vi "Actor Core.vi"(8 "error in (no error)":errorcluster, 11 "Waveform Plot.lvclass":refnum<class "Waveform Plot.lvclass">) -> (0 "error out":errorcluster, 3 "Actor out":refnum<class "Actor.lvclass">)   [LabVIEW 2015, in "Waveform Plot.lvclass"]
doc: "<B>Copyright:</B> (c) 2015 National Instruments. All rights reserved.\n\nOpens the .tdms file specified in the <B>file path</B> input and presents the file data in the TDMS File Viewer dialog box."
uses:
  Waveform Plot.lvclass
  Instance           1 26Saved   TDMS - File Viewer .vi
  <vilib>/Utility/tdmsutil.llb/fileViewerConfigData.ctl
  <vilib>/Utility/tdmsutil.llb/TDMSFileViewerLocalizedText.vi
  <vilib>/Utility/error.llb/DialogType.ctl
  <vilib>/event_ctls.llb/sizeaction.ctl
  <vilib>/event_ctls.llb/panelstate.ctl
  Plot/Plot.lvclass
  <vilib>/ActorFramework/Actor/Actor.lvclass
panel:
  out "LastXScaleFormat":u8
  out "TotalCount":u64
  out "Temp Configuration":T1
  in  "LastTopLeftValue":u64
  out "Resize?":bool
  in  "Help":bool
  out "file path out":path
  in  "Status":string
  in  "Settings...":bool
  in  "file path":path
  in  "Properties / Values / Graph":T2(tab)=enum."Analog values (graph)"
  in  "Properties":i32(listbox)
  in  "Quit":bool
  in  "Go To":bool
  in  "Scrollbar":u64(c297)
  in  "Raw data values":i32(listbox)
  out "Waveform Graph":waveform(dbl)[](graph)
  in  "File contents":string(tree)
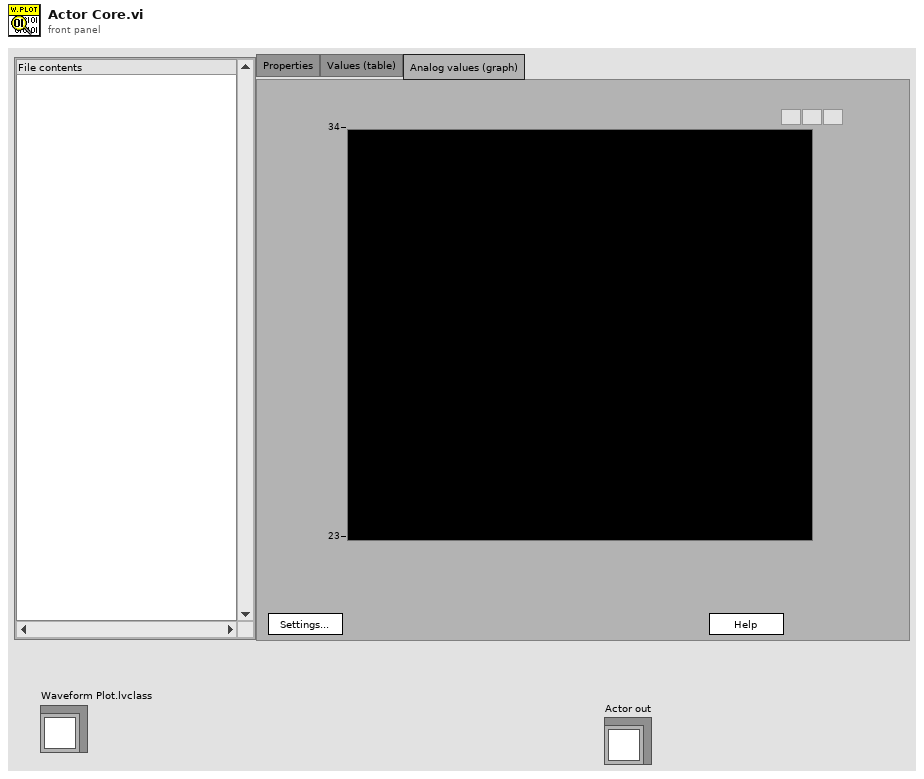
[diagram p1: front panel]
types:
  T1 = typedef "fileViewerConfigData.ctl" = cluster{"Show all (table)":bool, "Show all (graph)":bool, "limit (table)":u64, "limit (graph)":u64, "no show":bool, "start (table)":u64, "start (graph)":u64}
  T2 = enum32{"Properties", "Values (table)", "Analog values (graph)"}
  T3 = enum16{"open", "open or create", "create or replace", "create", "open (read-only)"}
  T4 = cluster{"Tree":refnum<vi>, "Tab Control":refnum<vi>, "property list":refnum<vi>, "raw data list":refnum<vi>, "Waveform Graph":refnum<vi>, "Ok":refnum<vi>, "Ok 2":refnum<vi>, "Ok 3":refnum<vi>, "Ok 4":refnum<vi>, "Scrollbar":refnum<vi>, "Ok 5":refnum<vi>, "TopLeftValue":refnum<vi>, "TotalCount":refnum<vi>}
  T5 = cluster{"File Path Control":path, "Group":string, "Channel":string, "Abbreviated":string}[]
  T6 = cluster{"File Path Control":path, "Group":string, "Channel":string, "Abbreviated":string}
  T7 = typedef "panelstate.ctl" = enum32{"Standard", "Minimized", "Maximized"}
  T8 = typedef "sizeaction.ctl" = enum32{"Minimized", "Maximized", "Resized"}
  T9 = cluster{"Shift":bool, "Ctrl":bool, "Alt":bool, "Cmd":bool, "Opt":bool}
  T10 = typedef "LVRectTypeDef.ctl" = cluster{"Left":i16, "Top":i16, "Right":i16, "Bottom":i16}
  T11 = typedef "LVRowAndColumnUnsignedTypeDef.ctl" = cluster{"Row":u32, "Column":u32}
  T12 = typedef "DialogType.ctl" = u16
  T13 = typedef "eventvkey.ctl" = enum16{"ASCII", "Enter", "Return", "Shift", "Ctrl", "Alt", "Cmd", "Opt", "Caps", "NumLock", "Clear", "Break", "Up", "Down", "Left", "Right", "Insert", "Delete", "Home", "End", "PageUp", "PageDown", "Escape", "Help", "Pause", "ScrollLock", "F1", "F2", "F3", "F4", "F5", "F6", "F7", "F8", "F9", "F10", "F11", "F12", "F13", "F14", "F15", "F16", "F17", "F18", "F19", "F20", "F21", "F22", "F23", "F24", "Play", "VolumeUp", "VolumeDown", "Mute", "Two Byte Char"}
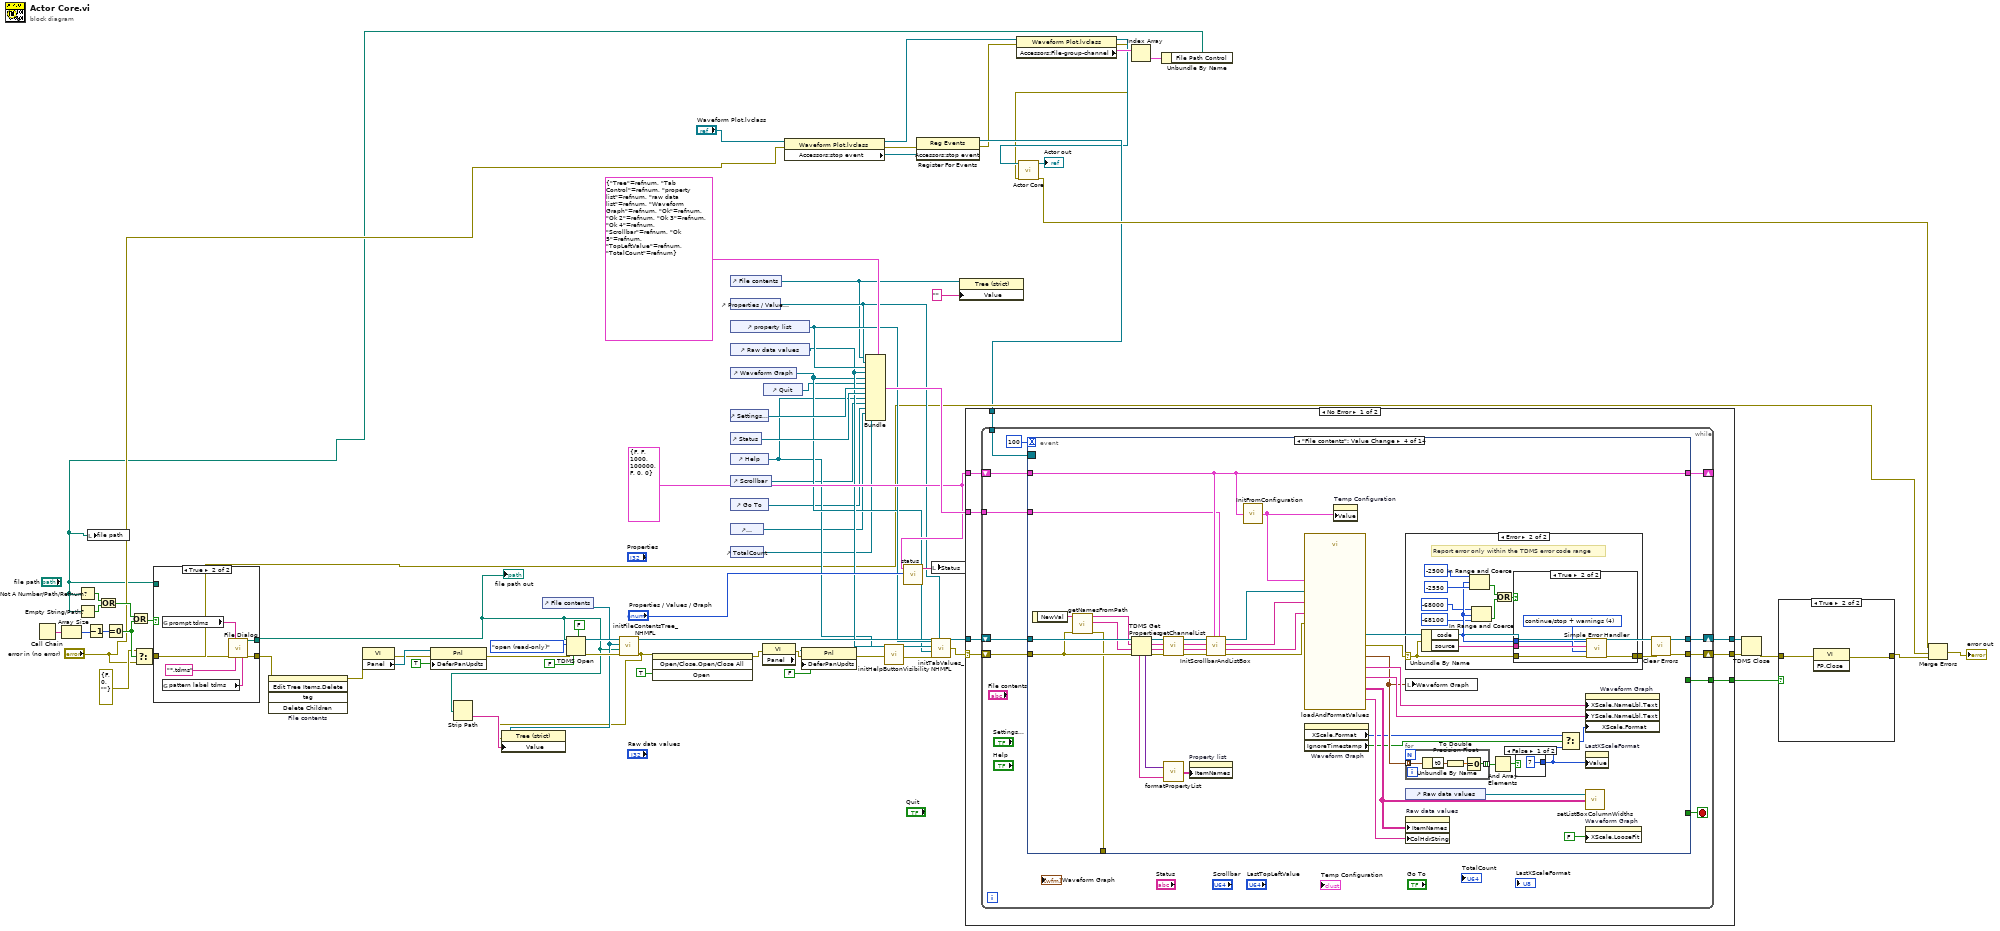
[diagram p0: block diagram]
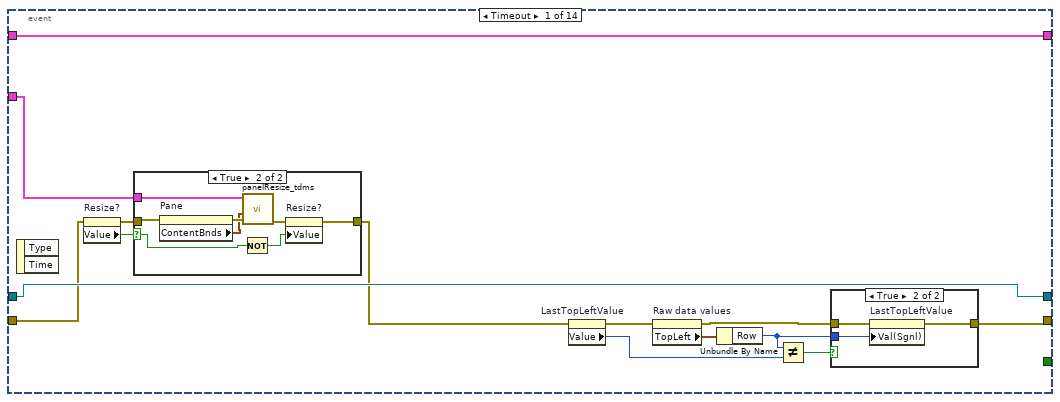
[diagram p3: hidden frame]
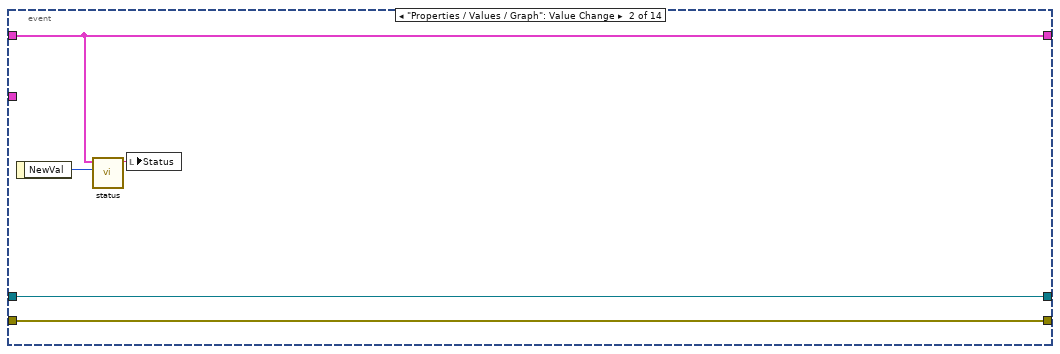
[diagram p6: hidden frame]
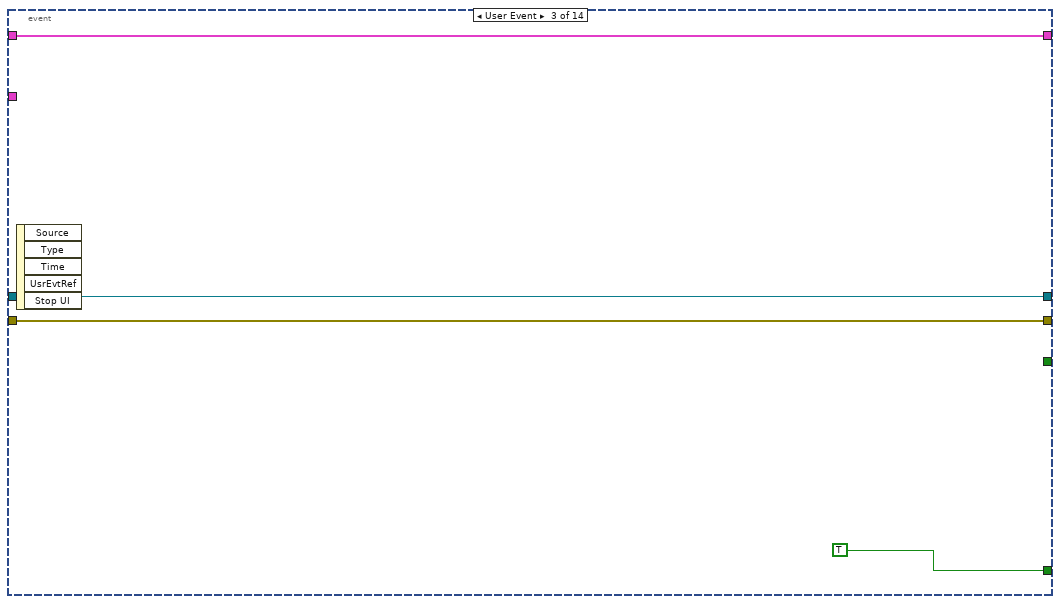
[diagram p7: hidden frame]
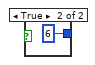
[diagram p8: hidden frame]
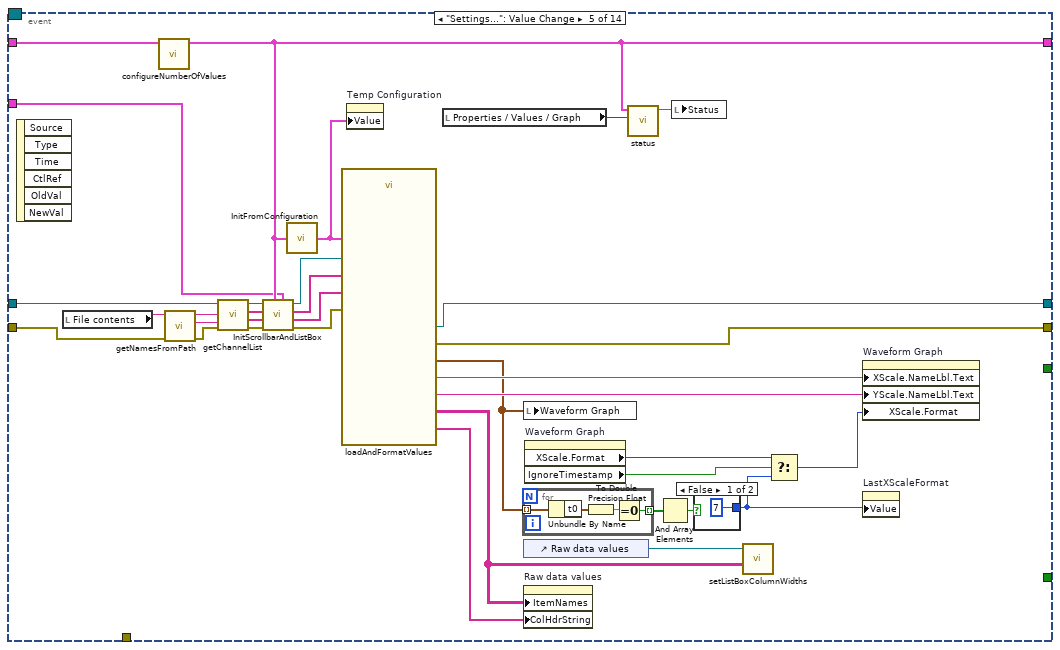
[diagram p11: hidden frame]
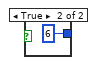
[diagram p12: hidden frame]
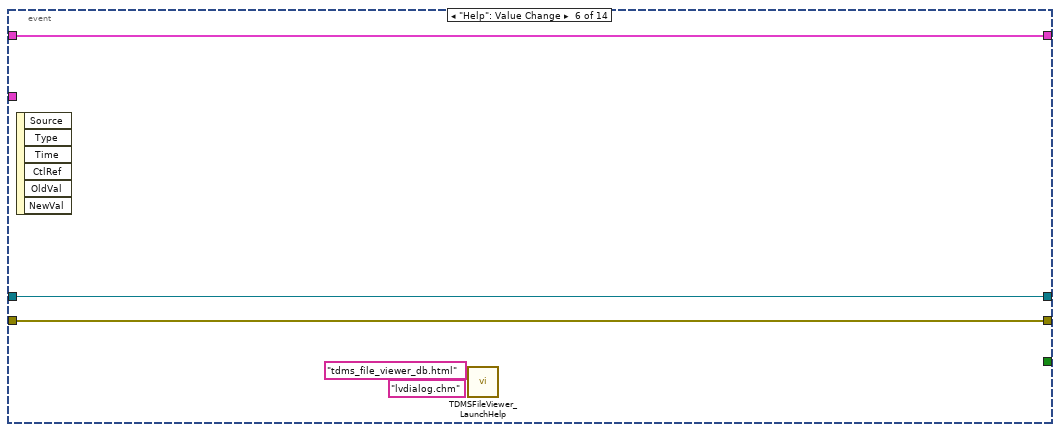
[diagram p13: hidden frame]
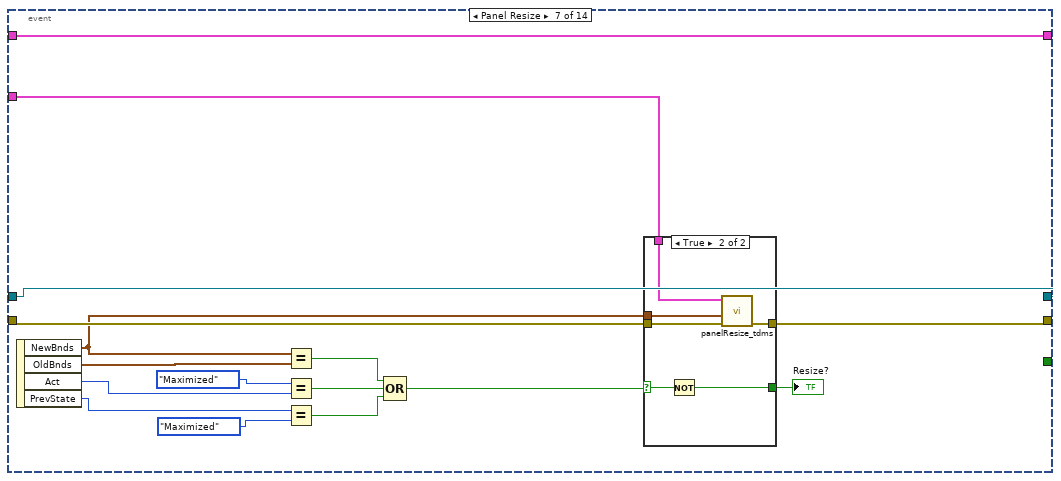
[diagram p14: hidden frame]
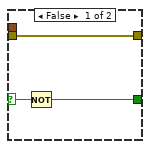
[diagram p15: hidden frame]
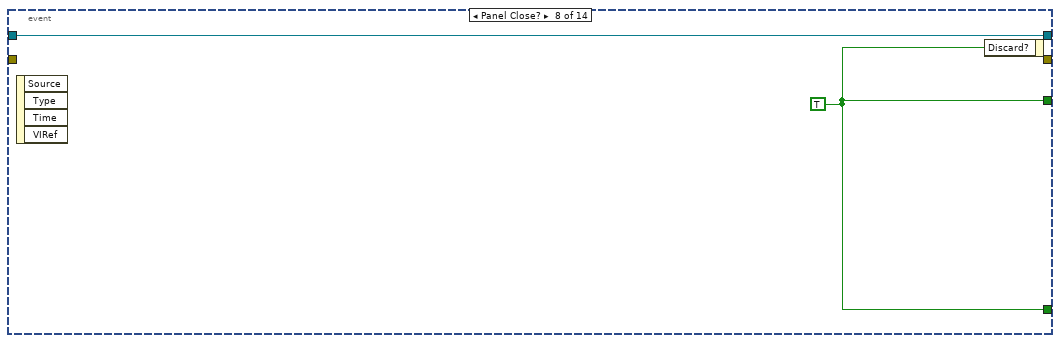
[diagram p16: hidden frame]
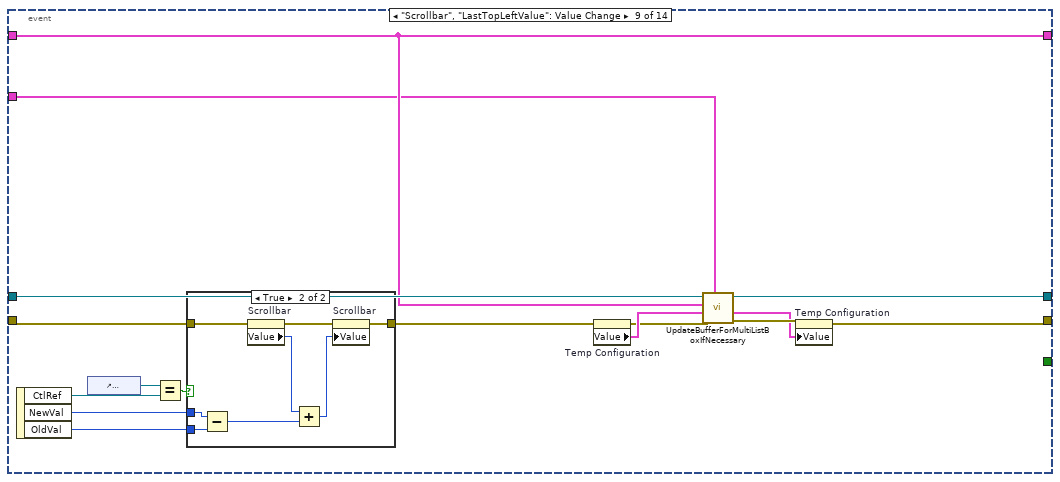
[diagram p17: hidden frame]
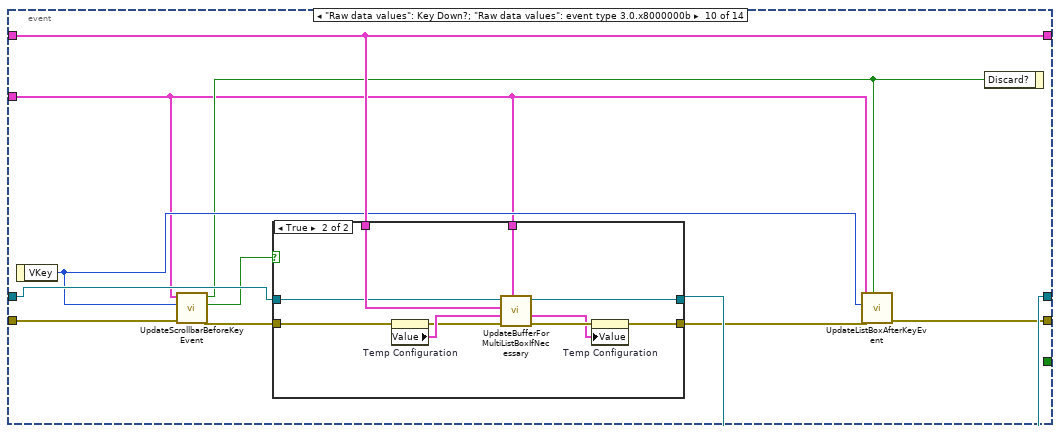
[diagram p19: hidden frame]
diagram:
  w44 = T1 {"Show all (table)"=FALSE, "Show all (graph)"=FALSE, "limit (table)"=1000, "limit (graph)"=100000, "no show"=FALSE, "start (table)"=0, "start (graph)"=0} ("TDMS File Viewer Configuration")
  n1 = Call Chain() -> (call chain=w56:string[])
  n2 = Array Size(array=w56) -> (size(s)=w54:i32)
  n3 = Decrement(x=w54) -> (x-1=w53:i32)
  n4 = Equal To 0?(x=w53) -> (x = 0?=w42:bool)
  n5 = Select(t=errorcluster {"status"=FALSE, "code"=0, "source"=""}, s=w42, f="error in (no error)") -> (s? t:f=w25:errorcluster)
  n6 = control-ref of="File contents"() -> (w4:refnum<vi>)
  n7 = control-ref of="File contents"() -> (w32:refnum<vi>)
  n8 = control-ref of="Properties / Values / Graph"() -> (w33:refnum<vi>)
  n9 = control-ref of="property list"() -> (w36:refnum<vi>)
  n10 = control-ref of="Raw data values"() -> (w35:refnum<vi>)
  n11 = control-ref of="Waveform Graph"() -> (w34:refnum<vi>)
  n12 = control-ref of="Settings..."() -> (w49:refnum<vi>)
  n13 = control-ref of="Status"() -> (w46:refnum<vi>)
  n14 = control-ref of="Help"() -> (w28:refnum<vi>)
  n15 = control-ref of="Scrollbar"() -> (w24:refnum<vi>)
  n16 = control-ref of="Go To"() -> (w23:refnum<vi>)
  n17 = control-ref of="LastTopLeftValue"() -> (w22:refnum<vi>)
  n18 = control-ref of="TotalCount"() -> (w21:refnum<vi>)
  n19 = control-ref of="Quit"() -> (w6:refnum<vi>)
  n20 = property class="Waveform Plot.lvclass"(reference="Waveform Plot.lvclass", error in="error in (no error)") -> (reference out=w10:refnum<class "Waveform Plot.lvclass">, error out=w15:errorcluster, "Accessors:stop event"=w14:refnum<user-event>)
  n21 = Bundle(cluster=T4 {"Tree"=refnum, "Tab Control"=refnum, "property list"=refnum, "raw data list"=refnum, "Waveform Graph"=refnum, "Ok"=refnum, "Ok 2"=refnum, "Ok 3"=refnum, "Ok 4"=refnum, "Scrollbar"=refnum, "Ok 5"=refnum, "TopLeftValue"=refnum, "TotalCount"=refnum} ("control refs"), "Tree"=w32, "Tab Control"=w33, "property list"=w36, "raw data list"=w35, "Waveform Graph"=w34, "Ok"=w6, "Ok 2"=w49, "Ok 3"=w46, "Ok 4"=w28, "Scrollbar"=w24, "Ok 5"=w23, "TopLeftValue"=w22, "TotalCount"=w21) -> (w51:T4)
  n22 = call <vilib>:"status.vi"("tab sheet"="Properties / Values / Graph", "TDMS File Viewer Configuration"=w44) -> ("status"=w45:string)  [unwired: 5 out]
  n23 = register-events(error in=w15, w14) -> (reference out=w13:refnum<event-registration>, error out=w8:errorcluster)  [unwired: 1 in]
  n24 = local write "Status"(w45) -> ()
  n25 = property class="Tree (strict)"(reference=w32, "Value"="") -> ()  [unwired: 1 in, 2 out]
  n26 = property class="Waveform Plot.lvclass"(reference=w10, error in=w8) -> (reference out=w9:refnum<class "Waveform Plot.lvclass">, error out=w7:errorcluster, "Accessors:File-group-channel"=w11:T5)
  n27 = call-parent "Actor Core.vi"("error in"=w7, "Measure Object in"=w9) -> ("error out"=w17:errorcluster, "Actor out"=→"Actor out":refnum<class "Actor.lvclass">)  [unwired: 8 in]
  n28 = Index Array(array=w11) -> (element=w12:T6)  [unwired: 1 in]
  n29 = Unbundle By Name(w12) -> ("File Path Control"=w5:path)
  n30 = Not A Number/Path/Refnum?(number/path/refnum=w5) -> (NaN/Path/Refnum?=w58:bool)
  n31 = Empty String/Path?(string/path=w5) -> (empty?=w57:bool)
  n32 = local write "file path"(w5) -> ()
  n33 = Or(x=w58, y=w57) -> (x .or. y?=w55:bool)
  n34 = Or(x=w55, y=w42) -> (x .or. y?=w52:bool)
  n35 = case shown="True" w52 {
    tunnel: [w75 w81] -> w3
    tunnel: w5 -> [w75 _]
    tunnel: [w74 w79] -> w47
    tunnel: w25 -> [w74 w78]
    frame False {
    }
    frame True {
      n36 = global read "TDMSFileViewerLocalizedText.vi" "prompt tdms"() -> (w77:string)
      n37 = global read "TDMSFileViewerLocalizedText.vi" "pattern label tdms"() -> (w76:string)
      n38 = call "File Dialog"("prompt"=w77, "error in"=w78, "pattern (all files)"="*.tdms", "pattern label"=w76) -> ("selected path"=w81:path, "error out"=w79:errorcluster)  [unwired: 3 in, 7 out]
    }
  }
  "file path out" <- w3
  n39 = invoke on="File contents" class="Tree (strict)" method="Edit Tree Items.Delete"(error in=w47) -> (error out=w64:errorcluster)  [unwired: 4 in, 4 out]
  n40 = property class="VI"(error in=w64) -> (error out=w65:errorcluster, "Panel"=w66:refnum<vi>)  [unwired: 1 in, 1 out]
  n41 = property class="Pnl"(reference=w66, error in=w65, "DeferPanUpdts"=TRUE ("Defer Panel Updates")) -> (error out=w68:errorcluster)  [unwired: 1 out]
  n42 = Strip Path(path=w3) -> (name=w2:string)  [unwired: 1 out]
  n43 = TDMS Open(5:FALSE ("create index file? (T)"), 6:FALSE ("disable buffering (T)"), 8:w68, 10:T3."open (read-only)" ("operation"), 11:w3) -> (0:w73:errorcluster, 3:w72:refnum<k34>)  [unwired: 2 in]
  n44 = call "initFileContentsTree_NHMFL.vi"("error in (no error)"=w73, "file path"=w3, "Tree Refnum"=w4, "tdms file"=w72) -> ("error out"=w1:errorcluster, "tdms file out"=w71:refnum<k34>)  [unwired: 2 out]
  n45 = property class="Tree (strict)"(reference=w4, error in=w1, "Value"=w2) -> ()  [unwired: 2 out]
  n46 = invoke on="File contents" class="Tree (strict)" method="Open/Close.Open/Close All"(error in=w1, "Open"=TRUE ("Open?")) -> (error out=w60:errorcluster)  [unwired: 2 in, 3 out]
  n47 = property class="VI"(error in=w60) -> (error out=w62:errorcluster, "Panel"=w61:refnum<vi>)  [unwired: 1 in, 1 out]
  n48 = property class="Pnl"(reference=w61, error in=w62, "DeferPanUpdts"=FALSE ("Defer Panel Updates")) -> (error out=w30:errorcluster)  [unwired: 1 out]
  n49 = call <vilib>:"initHelpButtonVisibility.vi"("error in"=w30, "Help"=w28) -> ("error out"=w29:errorcluster)  [unwired: 9 in]
  n50 = call "initTabValues_NHMFL.vi"("properties"=w36, "Values"=w35, "waveform"=w34, "error in"=w29, "Properties / Values / Graph"=w33) -> ("error out"=w37:errorcluster)
  n51 = case shown="No Error" w37 {
    selector: w37 -> [w84 w407]
    tunnel: w71 -> [w89 w408]
    tunnel: [w88 w408] -> w70
    tunnel: [w87 w406] -> w69
    tunnel: w51 -> [w86 _]
    tunnel: w44 -> [w85 _]
    tunnel: [w83 FALSE] -> w40
    tunnel: w13 -> [w82 _]
    frame No Error {
      n52 = while {
        shift-right: [w98] -> w87
        shift-left: w84 -> [w99]
        shift-right: [w97] -> w88
        shift-left: w89 -> [w100]
        tunnel: w86 -> [w95]
        shift-right: [w93] -> _
        shift-left: w85 -> [w94]
        tunnel: [w92] -> w83
        tunnel: w82 -> [w90]
        stop <- w96 stop-if-true
        n53 = event shown="[3] \"File contents\": Value Change" {
          selector: w90 -> [_ _ _ _ _ _ _ _ _ _ _ _ _ _]
          dyn-events: _ -> [_ _ _ _ _ _ _ _ _ _ _ _ _ _]
          timeout: 100 -> [_ _ _ _ _ _ _ _ _ _ _ _ _ _]
          tunnel: w100 -> [w114 w131 w135 w177 w225 w245 w262 w273 w289 w308 w333 w348 w381 w398]
          tunnel: w99 -> [w109 w132 w134 w169 w232 w244 w260 _ w276 w300 w322 w345 w380 w397]
          tunnel: [w102 w132 w134 w165 w233 w244 w259 _ w283 w305 w325 w346 w380 w389] -> w98
          tunnel: [w114 w131 w135 w176 w234 w245 w262 w273 w288 w307 w332 w347 w381 w398] -> w97
          tunnel: [_ _ TRUE ("Quit") _ _ _ _ w272 _ _ _ _ _ _] -> w96
          tunnel: [_ _ _ w168 _ _ _ _ _ _ _ _ _ _] -> _
          tunnel: w95 -> [w110 _ _ w144 w209 _ w261 _ w275 w301 w323 w342 _ _]
          tunnel: w94 -> [w113 w128 w133 w145 w235 w246 w258 _ w287 w309 w334 w349 w382 w399]
          tunnel: [w113 w128 w133 w145 w211 w246 w258 _ w287 w309 w334 w349 w382 w399] -> w93
          tunnel: [_ _ _ _ _ _ _ w272 _ _ _ _ _ _] -> w92
          event Timeout {
            n54 = event-data() -> ()  [unwired: 3 out]
            n55 = property on="Resize?" class="Bool (strict)"(error in=w109) -> (error out=w111:errorcluster, "Value"=w112:bool)  [unwired: 1 in, 1 out]
            n56 = case shown="True" w112 {
              selector: w112 -> [_ w126]
              tunnel: w110 -> [_ w127]
              tunnel: w111 -> [w119 w122]
              tunnel: [w119 w124] -> w107
              frame False {
              }
              frame True {
                n57 = property on="Pane" class="Pane"(error in=w122) -> (error out=w121:errorcluster, "ContentBnds"=w120:T10)  [unwired: 1 in, 1 out]
                n58 = Not(x=w126) -> (.not. x?=w123:bool)
                n59 = call <vilib>:"panelResize_tdms.vi"("error in (no error)"=w121, "NewBnds"=w120, "control refs"=w127) -> ("error out"=w125:errorcluster)  [unwired: 4 in]
                n60 = property on="Resize?" class="Bool (strict)"(error in=w125, "Value"=w123) -> (error out=w124:errorcluster)  [unwired: 1 in, 1 out]
              }
            }
            n61 = property on="LastTopLeftValue" class="DigNum (strict)"(error in=w107) -> (error out=w106:errorcluster, "Value"=w105:u64)  [unwired: 1 in, 1 out]
            n62 = property on="Raw data values" class="MCListbox (strict)"(error in=w106) -> (error out=w103:errorcluster, "TopLeft"=w108:T11)  [unwired: 1 in, 1 out]
            n63 = Unbundle By Name(w108) -> ("Row"=w101:u32)
            n64 = Not Equal?(x=w101, y=w105) -> (x != y?=w104:bool)
            n65 = case shown="True" w104 {
              tunnel: w103 -> [w115 w118]
              tunnel: [w115 w117] -> w102
              tunnel: w101 -> [_ w116]
              frame False {
              }
              frame True {
                n66 = property on="LastTopLeftValue" class="DigNum (strict)"(error in=w118, "Val(Sgnl)"=w116) -> (error out=w117:errorcluster)  [unwired: 1 in, 1 out]
              }
            }
          }
          event "Properties / Values / Graph": Value Change {
            n67 = event-data() -> ("NewVal"=w130:T2)  [unwired: 1 out]
            n68 = call <vilib>:"status.vi"("tab sheet"=w130, "TDMS File Viewer Configuration"=w128) -> ("status"=w129:string)  [unwired: 5 out]
            n69 = local write "Status"(w129) -> ()
          }
          event User Event {
            n70 = event-data() -> ()  [unwired: 6 out]
          }
          event "File contents": Value Change {
            n71 = event-data() -> ("NewVal"=w171:string)  [unwired: 1 out]
            n72 = call <vilib>:"getNamesFromPath.vi"("error in (no error)"=w169, "tree path"=w171) -> ("error out"=w168:errorcluster, "channel"=w174:string, "group"=w175:string)  [unwired: 3 out]
            n73 = TDMS Get Properties(8:w169, 9:w174, 10:w175, 11:w177) -> (0:w163:errorcluster, 1:w162:string, 2:w158:string, 3:w164:refnum<k34>, 4:w172:variant[], 6:w173:string[])  [unwired: 2 out]
            n74 = call <vilib>:"getChannelList.vi"("error in (no error)"=w163, "channel names"=w162, "group name"=w158, "tdms file"=w164) -> ("error out"=w153:errorcluster, "channel names out"=w151:string[], "group names out"=w149:string[], "tdms file out"=w147:refnum<k34>)
            n75 = call <vilib>:"formatPropertyList.vi"("property names"=w173, "property values"=w172) -> ("strings"=w170:string[][])
            n76 = property on="Property list" class="MCListbox (strict)"("ItemNames"=w170) -> ()  [unwired: 2 in, 2 out]
            n77 = call <vilib>:"InitScrollbarAndListBox.vi"("control refs"=w144, "configuration"=w145, "error in (no error)"=w153, "channel names"=w151, "group names"=w149, "tdms in"=w147) -> ("error out"=w152:errorcluster, "channel out"=w150:string[], "group out"=w148:string[], "tdms out"=w146:refnum<k34>)  [unwired: 2 in]
            n78 = call <vilib>:"InitFromConfiguration.vi"("configuration"=w145) -> ("output cluster"=w154:T1)  [unwired: 4 in]
            n79 = call <vilib>:"loadAndFormatValues.vi"("error in (no error)"=w152, "configuration"=w154, "channel names"=w150, "group names"=w148, "tdms file"=w146) -> ("error out"=w157:errorcluster, "graph y names"=w160:string, "graph x names"=w159:string, "tdms file out"=w176:refnum<k34>, "waveform values"=w143:waveform(dbl)[], "table values"=w167:string[][], "table headers"=w161:string[])
            n80 = property on="Waveform Graph" class="WFGraph (strict)"() -> ("XScale.Format"=w138:u8, "IgnoreTimestamp"=w137:bool)  [unwired: 2 in, 2 out]
            n81 = property on="Temp Configuration" class="Clust (strict)"("Value"=w154) -> ()  [unwired: 2 in, 2 out]
            n82 = case shown="Error" w157 {
              selector: w157 -> [w184 w194]
              tunnel: [w184 w193] -> w156
              frame No Error {
              }
              frame Error {
                # "Report error only within the TDMS error code range"
                n83 = Unbundle By Name(w194) -> ("code"=w190:i32, "source"=w195:string)
                n84 = In Range and Coerce(upper limit=-2500, x=w190, lower limit=-2550 ("upper limit")) -> (In Range?=w187:bool)  [unwired: 1 out]
                n85 = In Range and Coerce(upper limit=-68000, x=w190, lower limit=-68100) -> (In Range?=w186:bool)  [unwired: 1 out]
                n86 = Or(x=w187, y=w186) -> (x .or. y?=w185:bool)
                n87 = case shown="True" w185 {
                  tunnel: w195 -> [_ w201]
                  tunnel: w194 -> [w196 w200]
                  tunnel: [w196 w199] -> w193
                  tunnel: w190 -> [_ w197]
                  frame False {
                    # "Out of the range of TDMS\nerror code, we don't report\nthem."
                  }
                  frame True {
                    w198 = T12 4 items=["no dialog", "OK message", "continue or stop message", "OK message + warnings", "continue/stop + warnings"] ("type of dialog (OK msg:1)")
                    n88 = call <vilib>:"Simple Error Handler.vi"("error code (no error:0)"=w197, "error source (\" \")"=w201, "type of dialog (OK msg:1)"=w198, "error in (no error)"=w200) -> ("error out"=w199:errorcluster)  [unwired: 1 in, 4 out]
                  }
                }
              }
            }
            n89 = local write "Waveform Graph"(w143) -> ()
            n90 = for {
              tunnel: w143 -> [w183] mode=indexing
              tunnel: [w180] -> w142 mode=indexing
              n91 = Unbundle By Name(w183) -> ("t0"=w182:timestamp)
              n92 = To Double Precision Float(number=w182) -> (double precision float=w181:dbl)
              n93 = Equal To 0?(x=w181) -> (x = 0?=w180:bool)
            }
            n94 = control-ref of="Raw data values"() -> (w166:refnum<vi>)
            n95 = property on="Raw data values" class="MCListbox (strict)"("ItemNames"=w167, "ColHdrString"=w161) -> ()  [unwired: 2 in, 2 out]
            n96 = And Array Elements(Boolean array=w142) -> (logical AND=w141:bool)
            n97 = case shown="False" w141 {
              tunnel: [u8 7 u8 6] -> w139
              frame False {
              }
              frame True {
              }
            }
            n98 = Select(t=w138, s=w137, f=w139) -> (s? t:f=w140:u8)
            n99 = property on="Waveform Graph" class="WFGraph (strict)"("XScale.NameLbl.Text"=w159, "YScale.NameLbl.Text"=w160, "XScale.Format"=w140) -> ()  [unwired: 2 in, 2 out]
            n100 = property on="LastXScaleFormat" class="DigNum (strict)"("Value"=w139) -> ()  [unwired: 2 in, 2 out]
            n101 = call <vilib>:"setListBoxColumnWidths.vi"("table data"=w167, "MCListbox Refnum"=w166) -> ()  [unwired: 1 out]
            n102 = property on="Waveform Graph" class="WFGraph (strict)"("XScale.LooseFit"=FALSE ("X Scale.Loose Fit")) -> ()  [unwired: 2 in, 2 out]
            n103 = call <vilib>:"Clear Errors.vi"("error in (no error)"=w156) -> ("error out"=w165:errorcluster)  [unwired: 1 in, 5 out]
          }
          event "Settings...": Value Change {
            n104 = event-data() -> ()  [unwired: 7 out]
            n105 = local read "File contents"() -> (w226:string)
            n106 = call <vilib>:"configureNumberOfValues.vi"("TDMS File Viewer Configuration"=w235) -> ("TDMS File Viewer Configuration Out"=w211:T1)  [unwired: 10 out]
            n107 = call <vilib>:"getNamesFromPath.vi"("error in (no error)"=w232, "tree path"=w226) -> ("error out"=w224:errorcluster, "channel"=w222:string, "group"=w223:string)  [unwired: 3 out]
            n108 = call <vilib>:"getChannelList.vi"("error in (no error)"=w224, "channel names"=w222, "group name"=w223, "tdms file"=w225) -> ("error out"=w213:errorcluster, "channel names out"=w215:string[], "group names out"=w217:string[], "tdms file out"=w219:refnum<k34>)
            n109 = call <vilib>:"InitScrollbarAndListBox.vi"("control refs"=w209, "configuration"=w211, "error in (no error)"=w213, "channel names"=w215, "group names"=w217, "tdms in"=w219) -> ("error out"=w212:errorcluster, "channel out"=w214:string[], "group out"=w216:string[], "tdms out"=w218:refnum<k34>)  [unwired: 2 in]
            n110 = call <vilib>:"InitFromConfiguration.vi"("configuration"=w211) -> ("output cluster"=w210:T1)  [unwired: 4 in]
            n111 = call <vilib>:"loadAndFormatValues.vi"("error in (no error)"=w212, "configuration"=w210, "channel names"=w214, "group names"=w216, "tdms file"=w218) -> ("error out"=w233:errorcluster, "graph y names"=w228:string, "graph x names"=w227:string, "tdms file out"=w234:refnum<k34>, "waveform values"=w206:waveform(dbl)[], "table values"=w229:string[][], "table headers"=w231:string[])
            n112 = property on="Temp Configuration" class="Clust (strict)"("Value"=w210) -> ()  [unwired: 2 in, 2 out]
            n113 = local read "Properties / Values / Graph"() -> (w220:T2)
            n114 = for {
              tunnel: w206 -> [w241] mode=indexing
              tunnel: [w238] -> w208 mode=indexing
              n115 = Unbundle By Name(w241) -> ("t0"=w240:timestamp)
              n116 = To Double Precision Float(number=w240) -> (double precision float=w239:dbl)
              n117 = Equal To 0?(x=w239) -> (x = 0?=w238:bool)
            }
            n118 = local write "Waveform Graph"(w206) -> ()
            n119 = control-ref of="Raw data values"() -> (w230:refnum<vi>)
            n120 = property on="Raw data values" class="MCListbox (strict)"("ItemNames"=w229, "ColHdrString"=w231) -> ()  [unwired: 2 in, 2 out]
            n121 = property on="Waveform Graph" class="WFGraph (strict)"() -> ("XScale.Format"=w203:u8, "IgnoreTimestamp"=w202:bool)  [unwired: 2 in, 2 out]
            n122 = call <vilib>:"status.vi"("tab sheet"=w220, "TDMS File Viewer Configuration"=w211) -> ("status"=w221:string)  [unwired: 5 out]
            n123 = And Array Elements(Boolean array=w208) -> (logical AND=w207:bool)
            n124 = local write "Status"(w221) -> ()
            n125 = case shown="False" w207 {
              tunnel: [u8 7 u8 6] -> w204
              frame False {
              }
              frame True {
              }
            }
            n126 = call <vilib>:"setListBoxColumnWidths.vi"("table data"=w229, "MCListbox Refnum"=w230) -> ()  [unwired: 1 out]
            n127 = Select(t=w203, s=w202, f=w204) -> (s? t:f=w205:u8)
            n128 = property on="Waveform Graph" class="WFGraph (strict)"("XScale.NameLbl.Text"=w227, "YScale.NameLbl.Text"=w228, "XScale.Format"=w205) -> ()  [unwired: 2 in, 2 out]
            n129 = property on="LastXScaleFormat" class="DigNum (strict)"("Value"=w204) -> ()  [unwired: 2 in, 2 out]
          }
          event "Help": Value Change {
            n130 = event-data() -> ()  [unwired: 7 out]
            n131 = call <vilib>:"TDMSFileViewer_LaunchHelp.vi"("CHM or HLP filename (lvdialog.chm)"="lvdialog.chm", "HTML filename"="tdms_file_viewer_db.html") -> ()  [unwired: 1 in, 5 out]
          }
          event Panel Resize {
            n132 = event-data() -> ("NewBnds"=w250:T10, "OldBnds"=w249:T10, "Act"=w251:T8, "PrevState"=w252:T7)  [unwired: 1 out]
            n133 = Equal?(x=w250, y=w249) -> (x = y?=w255:bool)
            n134 = Equal?(x=sizeaction."Maximized" ("Act"), y=w251) -> (x = y?=w254:bool)
            n135 = Equal?(x=w252, y=panelstate."Maximized" ("PrevState")) -> (x = y?=w253:bool)
            n136 = Compound Arithmetic op=OR(w255, w254, w253) -> (w248:bool)
            n137 = case shown="True" w248 {
              selector: w248 -> [w264 w267]
              tunnel: w261 -> [_ w271]
              tunnel: w260 -> [w265 w270]
              tunnel: [w265 w269] -> w259
              tunnel: w250 -> [_ w268]
              tunnel: [w263 w266] -> w247
              frame False {
                n138 = Not(x=w264) -> (.not. x?=w263:bool)
              }
              frame True {
                n139 = Not(x=w267) -> (.not. x?=w266:bool)
                n140 = call <vilib>:"panelResize_tdms.vi"("error in (no error)"=w270, "NewBnds"=w268, "control refs"=w271) -> ("error out"=w269:errorcluster)  [unwired: 4 in]
              }
            }
            "Resize?" <- w247
          }
          event Panel Close? {
            w272 = TRUE
            n141 = event-data() -> ()  [unwired: 5 out]
            n142 = event-data("Discard?"=w272) -> ()  [unwired: 1 in, 1 out]
          }
          event "Scrollbar", "LastTopLeftValue": Value Change {
            n143 = event-data() -> ("CtlRef"=w281:refnum<vi>, "NewVal"=w278:u64, "OldVal"=w277:u64)  [unwired: 1 out]
            n144 = control-ref of="LastTopLeftValue"() -> (w280:refnum<vi>)
            n145 = Equal?(x=w280, y=w281) -> (x = y?=w279:bool)
            n146 = case shown="True" w279 {
              tunnel: w278 -> [_ w294]
              tunnel: w277 -> [_ w293]
              tunnel: w276 -> [w290 w292]
              tunnel: [w290 w291] -> w274
              frame False {
              }
              frame True {
                n147 = Subtract(x=w294, y=w293) -> (x-y=w296:u64)
                n148 = property on="Scrollbar" class="Scroll (strict)"(error in=w292) -> (error out=w298:errorcluster, "Value"=w297:u64)  [unwired: 1 in, 1 out]
                n149 = Add(x=w297, y=w296) -> (x+y=w295:u64)
                n150 = property on="Scrollbar" class="Scroll (strict)"(error in=w298, "Value"=w295) -> (error out=w291:errorcluster)  [unwired: 1 in, 1 out]
              }
            }
            n151 = property on="Temp Configuration" class="Clust (strict)"(error in=w274) -> (error out=w285:errorcluster, "Value"=w286:T1)  [unwired: 1 in, 1 out]
            n152 = call <vilib>:"UpdateBufferForMultiListBoxIfNecessary.vi"("control refs"=w275, "error in"=w285, "Buffer Configuration"=w286, "TDMS File Viewer Configuration"=w287, "tdms file in"=w289) -> ("error out"=w284:errorcluster, "BufferConfig out"=w282:T1, "tdms file out"=w288:refnum<k34>)  [unwired: 4 in]
            n153 = property on="Temp Configuration" class="Clust (strict)"(error in=w284, "Value"=w282) -> (error out=w283:errorcluster)  [unwired: 1 in, 1 out]
          }
          event "Raw data values": Key Down?; "Raw data values": event type 3.0.x8000000b {
            n154 = event-data() -> ("VKey"=w303:T13)  [unwired: 1 out]
            n155 = call <vilib>:"UpdateScrollbarBeforeKeyEvent.vi"("error in (no error)"=w300, "VKey"=w303, "control refs 2"=w301) -> ("error out"=w306:errorcluster, "LoadBuffer?"=w304:bool, "DiscardEvent?"=w302:bool)  [unwired: 6 in]
            n156 = case shown="True" w304 {
              tunnel: w309 -> [_ w317]
              tunnel: w308 -> [w310 w316]
              tunnel: [w310 w315] -> w307
              tunnel: w306 -> [w311 w312]
              tunnel: [w311 w314] -> w299
              tunnel: w301 -> [_ w313]
              frame False {
              }
              frame True {
                n157 = property on="Temp Configuration" class="Clust (strict)"(error in=w312) -> (error out=w320:errorcluster, "Value"=w321:T1)  [unwired: 1 in, 1 out]
                n158 = call <vilib>:"UpdateBufferForMultiListBoxIfNecessary.vi"("control refs"=w313, "error in"=w320, "Buffer Configuration"=w321, "TDMS File Viewer Configuration"=w317, "tdms file in"=w316) -> ("error out"=w319:errorcluster, "BufferConfig out"=w318:T1, "tdms file out"=w315:refnum<k34>)  [unwired: 4 in]
                n159 = property on="Temp Configuration" class="Clust (strict)"(error in=w319, "Value"=w318) -> (error out=w314:errorcluster)  [unwired: 1 in, 1 out]
              }
            }
            n160 = call <vilib>:"UpdateListBoxAfterKeyEvent.vi"("DiscardEvent?"=w302, "error in (no error)"=w299, "VKey"=w303, "control refs"=w301) -> ("error out"=w305:errorcluster)  [unwired: 7 in]
            n161 = event-data("Discard?"=w302) -> ()  [unwired: 1 in, 1 out]
          }
          event "Go To": Value Change {
            n162 = event-data() -> ()  [unwired: 2 out]
            n163 = call <vilib>:"GoTo.vi"("error in"=w322, "control refs"=w323) -> ("error out"=w331:errorcluster, "VisibleValue"=w328:u64)  [unwired: 8 in]
            n164 = property on="Temp Configuration" class="Clust (strict)"(error in=w331) -> (error out=w337:errorcluster, "Value"=w338:T1)  [unwired: 1 in, 1 out]
            n165 = call <vilib>:"UpdateBufferForMultiListBoxIfNecessary.vi"("control refs"=w323, "error in"=w337, "Buffer Configuration"=w338, "TDMS File Viewer Configuration"=w334, "tdms file in"=w333) -> ("error out"=w336:errorcluster, "BufferConfig out"=w335:T1, "tdms file out"=w332:refnum<k34>)  [unwired: 4 in]
            n166 = property on="Temp Configuration" class="Clust (strict)"(error in=w336, "Value"=w335) -> (error out=w324:errorcluster)  [unwired: 1 in, 1 out]
            n167 = property on="Raw data values" class="MCListbox (strict)"(error in=w324) -> (error out=w326:errorcluster, "TopLeft"=w330:T11)  [unwired: 1 in, 1 out]
            n168 = Unbundle By Name(w330) -> ("Row"=w329:u32)
            n169 = Add(x=w329, y=w328) -> (x+y=w327:u64)
            n170 = property on="Raw data values" class="MCListbox (strict)"(error in=w326, "Value"=w327) -> (error out=w325:errorcluster)  [unwired: 1 in, 1 out]
          }
          event Key Down {
            n171 = event-data() -> ("PlatMods"=w341:T9, "Char"=w340:i16)  [unwired: 1 out]
            n172 = property on="Raw data values" class="MCListbox (strict)"(error in=w345) -> (error out=w339:errorcluster, "Key Focus"=w344:bool)  [unwired: 1 in, 1 out]
            n173 = case shown="True" w344 {
              selector: w344 -> [w350 _]
              tunnel: [w350 w351] -> w343
              tunnel: w341 -> [_ w356]
              tunnel: w340 -> [_ w355]
              frame False {
              }
              frame True {
                n174 = disable-structure shown="Default" {
                  disable-tunnel: [T9 {"Shift"=FALSE, "Ctrl"=TRUE, "Alt"=FALSE, "Cmd"=FALSE, "Opt"=TRUE} ("PlatMods") T9 {"Shift"=FALSE, "Ctrl"=FALSE, "Alt"=FALSE, "Cmd"=TRUE, "Opt"=FALSE} ("PlatMods")] -> w357
                  frame condition #0 (active) {
                  }
                  frame condition #1 {
                  }
                }
                n175 = Equal?(x=w357, y=w356) -> (x = y?=w353:bool)
                n176 = Equal?(x=w355, y=i16 103 ("Char")) -> (x = y?=w352:bool)
                n177 = And(x=w353, y=w352) -> (x .and. y?=w351:bool)
              }
            }
            n178 = case shown="True" w343 {
              tunnel: w349 -> [_ w375]
              tunnel: w348 -> [w360 w374]
              tunnel: [w360 w373] -> w347
              tunnel: [w361 w366] -> w346
              tunnel: w339 -> [w361 w362]
              tunnel: w342 -> [_ w364]
              tunnel: w342 -> [_ w363]
              frame False {
              }
              frame True {
                n179 = call <vilib>:"GoTo.vi"("error in"=w362, "control refs"=w363) -> ("error out"=w372:errorcluster, "VisibleValue"=w369:u64)  [unwired: 8 in]
                n180 = property on="Temp Configuration" class="Clust (strict)"(error in=w372) -> (error out=w378:errorcluster, "Value"=w379:T1)  [unwired: 1 in, 1 out]
                n181 = call <vilib>:"UpdateBufferForMultiListBoxIfNecessary.vi"("control refs"=w364, "error in"=w378, "Buffer Configuration"=w379, "TDMS File Viewer Configuration"=w375, "tdms file in"=w374) -> ("error out"=w377:errorcluster, "BufferConfig out"=w376:T1, "tdms file out"=w373:refnum<k34>)  [unwired: 4 in]
                n182 = property on="Temp Configuration" class="Clust (strict)"(error in=w377, "Value"=w376) -> (error out=w365:errorcluster)  [unwired: 1 in, 1 out]
                n183 = property on="Raw data values" class="MCListbox (strict)"(error in=w365) -> (error out=w367:errorcluster, "TopLeft"=w371:T11)  [unwired: 1 in, 1 out]
                n184 = Unbundle By Name(w371) -> ("Row"=w370:u32)
                n185 = Add(x=w370, y=w369) -> (x+y=w368:u64)
                n186 = property on="Raw data values" class="MCListbox (strict)"(error in=w367, "Value"=w368) -> (error out=w366:errorcluster)  [unwired: 1 in, 1 out]
              }
            }
          }
          event Key Down? {
            n187 = event-data() -> ("VKey"=w384:T13)  [unwired: 1 out]
            n188 = case shown="\"F1\"" w384 {
              tunnel: [FALSE ("Discard?") TRUE ("Discard?")] -> w383
              frame Default {
              }
              frame "F1" {
                n189 = call <vilib>:"TDMSFileViewer_LaunchHelp.vi"("CHM or HLP filename (lvdialog.chm)"="lvdialog.chm", "HTML filename"="tdms_file_viewer_db.html") -> ()  [unwired: 1 in, 5 out]
              }
            }
            n190 = event-data("Discard?"=w383) -> ()  [unwired: 1 in, 1 out]
          }
          event "Waveform Graph": Shortcut Menu Selection (App) {
            n191 = event-data() -> ("ItemTag"=w395:string)  [unwired: 1 out]
            n192 = property on="Waveform Graph" class="WFGraph (strict)"(error in=w397) -> (error out=w390:errorcluster, "IgnoreTimestamp"=w394:bool)  [unwired: 1 in, 1 out]
            n193 = Not(x=w394) -> (.not. x?=w391:bool)
            n194 = Equal?(x=w395, y="APP_SC_IGNORE_TIME_STAMP") -> (x = y?=w392:bool)
            n195 = And(x=w391, y=w392) -> (x .and. y?=w393:bool)
            n196 = case shown="True" w393 {
              tunnel: w390 -> [w400 w404]
              tunnel: [w400 w401] -> w389
              frame False {
              }
              frame True {
                n197 = property on="LastXScaleFormat" class="DigNum (strict)"(error in=w404) -> (error out=w403:errorcluster, "Value"=w402:u8)  [unwired: 1 in, 1 out]
                n198 = property on="Waveform Graph" class="WFGraph (strict)"(error in=w403, "XScale.Format"=w402) -> (error out=w401:errorcluster)  [unwired: 1 in, 1 out]
              }
            }
          }
        }
      }
    }
    frame Error {
      n199 = call <vilib>:"Simple Error Handler.vi"("error in (no error)"=w407) -> ("error out"=w406:errorcluster)  [unwired: 1 in, 7 out]
    }
  }
  n200 = TDMS Close(8:w69, 11:w70) -> (0:w39:errorcluster)  [unwired: 1 out]
  n201 = case shown="True" w40 {
    tunnel: w39 -> [w409 w411]
    tunnel: [w409 w410] -> w27
    frame False {
    }
    frame True {
      n202 = invoke class="VI" method="FP.Close"(error in=w411) -> (error out=w410:errorcluster)  [unwired: 2 in, 2 out]
    }
  }
  n203 = Merge Errors(w17, w25, w27) -> (→"error out":errorcluster)
